vi "Write Items.vi"(8 "error in (no error)":errorcluster, 10 "Items":T1(array[cluster]), 11 "FSM.Annotation in":refnum<class "FSM.Annotation.lvclass">) -> (0 "error out":errorcluster, 3 "FSM.Annotation out":refnum<class "FSM.Annotation.lvclass">)   [LabVIEW 2020, in "FSM.Annotation.lvclass"]
uses:
  FSM.Annotation.lvclass
  FSM.Annotation.lvclass/FSM.Annotation.ctl
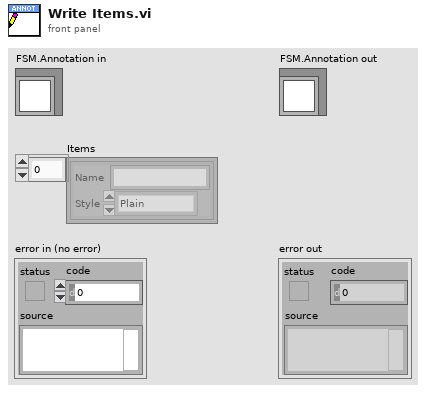
[diagram p1: front panel]
types:
  T1 = cluster{"Name":string, "Style":enum16{"Plain", "On", "Off", "On-Off"}}[]
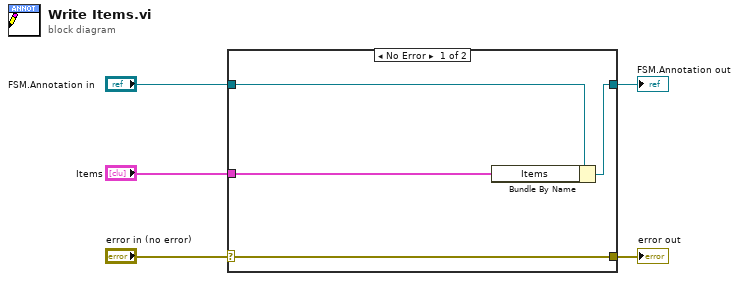
[diagram p0: block diagram]
diagram:
  n1 = case shown="No Error" "error in (no error)" {
    selector: "error in (no error)" -> [w9 w10]
    tunnel: [w9 w10] -> w4
    tunnel: [w7 w11] -> w2
    tunnel: "FSM.Annotation in" -> [w8 w11]
    tunnel: "Items" -> [w6 _]
    frame No Error {
      n2 = Bundle By Name(cluster=w8, "Items"=w6) -> (w7:refnum<class "FSM.Annotation.lvclass">)
    }
    frame Error {
    }
  }
  "error out" <- w4
  "FSM.Annotation out" <- w2
